vi "Disconnect Channels (Single).vi"(8 "error in (no error)":errorcluster, 9 "channel 2":string, 10 "channel 1":string, 11 "SLSC Switch in":refnum<class "SLSC Switch.lvclass">) -> (0 "error out":errorcluster, 3 "SLSC Switch out":refnum<class "SLSC Switch.lvclass">)   [LabVIEW 2015, in "SLSC Switch.lvclass"]
uses:
  SLSC Switch.lvclass
  SLSC Switch.lvclass/SLSC Switch.ctl
  Route Manager/Route Manager.lvclass
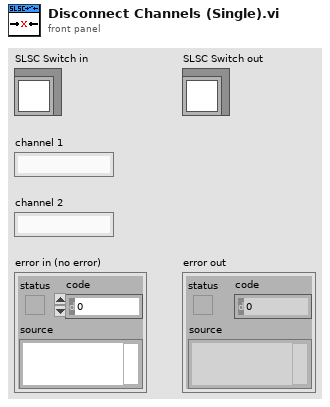
[diagram p1: front panel]
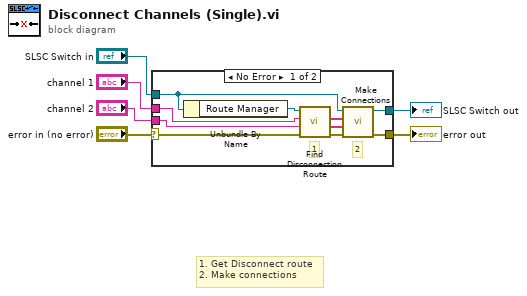
[diagram p0: block diagram]
diagram:
  # "1. Get Disconnect route\n2. Make connections"
  n1 = case shown="No Error" "error in (no error)" {
    selector: "error in (no error)" -> [w13 w18]
    tunnel: [w7 w18] -> w5
    tunnel: [w11 w17] -> w3
    tunnel: "SLSC Switch in" -> [w12 w17]
    tunnel: "channel 1" -> [w15 _]
    tunnel: "channel 2" -> [w14 _]
    frame No Error {
      # "2"
      # "1"
      n2 = Unbundle By Name(w12) -> ("Route Manager"=w16:refnum<class "Route Manager.lvclass">)
      n3 = call "Find Disconnection Route.vi"("error in (no error)"=w13, "channel 2"=w14, "channel 1"=w15, "Route Manager in"=w16) -> ("error out"=w8:errorcluster, "relays to close"=w9:string[], "relays to open"=w10:string[])  [unwired: 5 in]
      n4 = call "Make Connections.vi"("error in (no error)"=w8, "relays to close"=w9, "relays to open"=w10, "SLSC Switch in"=w12) -> ("error out"=w7:errorcluster, "SLSC Switch out"=w11:refnum<class "SLSC Switch.lvclass">)  [unwired: 6 in]
    }
    frame Error {
    }
  }
  "error out" <- w5
  "SLSC Switch out" <- w3
